vi "Open EXE.vi"(8 "error in (no error)":errorcluster, 10 "Build specification name":string, 11 "Project Refnum":refnum<vi>) -> (0 "error out":errorcluster, 3 "EXE out":refnum<class "NI_AB_API_EXE.lvclass">)   [LabVIEW 2020, in "NI_AB_API_EXE.lvclass"]
uses:
  <vilib>/AppBuilder/AB_API/EXE/NI_AB_API_EXE.lvclass
  e:/builds/penguin/labview/branches/2020/dev/dist/vi.lib/AppBuilder/AB_API/Build/NI_AB_API_Build.lvclass
  <vilib>/AppBuilder/AB_API/common/AB_API Build Object Type.ctl
  <vilib>/AppBuilder/AB_Classes/Build/AB_Build.lvclass
  <vilib>/AppBuilder/AB_API/Build/NI_AB_API_Build.lvclass
panel:
  in  "TargetItem Refnum":refnum<vi>
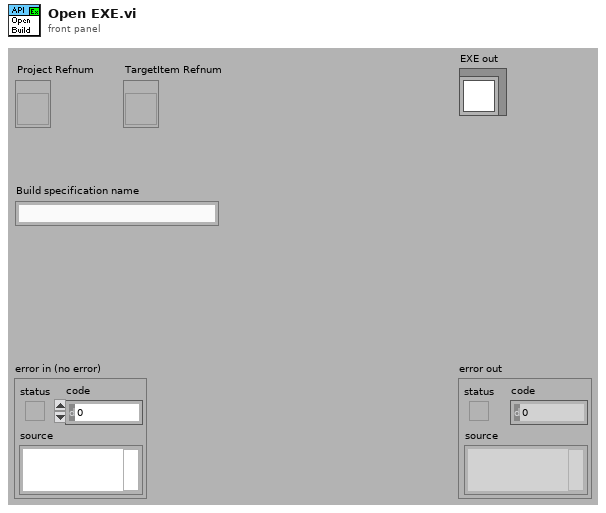
[diagram p1: front panel]
types:
  T1 = typedef "AB_API Build Object Type.ctl" = enum16{"Source Distribution", "DLL", "EXE", "Installer", "Zip File", "RESTful WS", "RTEXE", "Packed Library", "C Generation ", ".NET Interop Assembly"}
  T2 = typedef "ItemRef.ctl" = u64
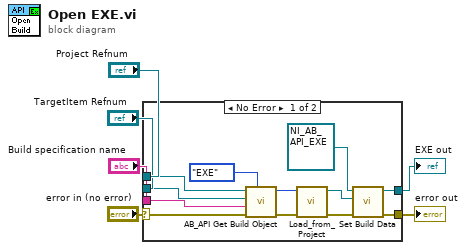
[diagram p0: block diagram]
diagram:
  n1 = case shown="No Error" "error in (no error)" {
    selector: "error in (no error)" -> [w12 w19]
    tunnel: [w8 w19] -> w5
    tunnel: [w10 _] -> w4
    tunnel: "Project Refnum" -> [w15 _]
    tunnel: "TargetItem Refnum" -> [w14 _]
    tunnel: "Build specification name" -> [w13 _]
    frame No Error {
      n2 = call <vilib>:"AB_API Get Build Object.vi"("Build object type"=AB_API_Build_Object_Type."EXE", "error in (no error)"=w12, "Build spec name"=w13, "TargetItem Refnum"=w14, "Project Refnum"=w15) -> ("error out"=w16:errorcluster, "Build Object"=w17:T2)  [unwired: 5 out]
      n3 = call <vilib>:"Load_from_Project.vi"("error in (no error)"=w16, "Object"=w17) -> ("error out"=w9:errorcluster, "Build out"=w7:refnum<class "AB_Build.lvclass">)  [unwired: 8 out]
      n4 = call <vilib>:"Set Build Data.vi"("error in (no error)"=w9, "AB_Build.lvclass"=w7, "NI_AB_API_Build in"=refnum<class "NI_AB_API_EXE.lvclass"> refnum ("NI_AB_API_DLL.lvclass")) -> ("error out"=w8:errorcluster, "NI_AB_API_Build out"=w10:refnum<class "NI_AB_API_EXE.lvclass">)  [unwired: 7 in]
    }
    frame Error {
    }
  }
  "error out" <- w5
  "EXE out" <- w4
